vi "ProdaNG.TestValues.Get.vi"(8 "error in (no error)":errorcluster, 10 "testStepId":i32, 11 "dbHandleIn":i32) -> (0 "error out":errorcluster, 2 "TestStepValues":T1[](array[typedef]) {"minimum" format="%#.3f"; "maximum" format="%#.3f"}, 3 "dbHandle":i32)   [LabVIEW 2016]
doc: "This function returns a product structure for a product, which is identified by a part and a serial number.\nImportant information: The field 'individual' was taken over from the field 'allgemein' of the legacy data directly. Because of this most products have the value 0 further on and only a few the value 1. \nParameter:\nhandle is an Integer, which is returned by the function Login() at the creation of a new connection.\nwabcoPartId is the Id of the part.\nserialNumber is the serial number of the product for the part above.\nproduct is a pointer on a product structure, which is filled if the returncode is 0. The structure must be defined in the calling program.\n\nReturncodes:\n0 No error\n< 0 ORACLE Error code\n6 (ERROR_INVALID_HANDLE) in case of an invalid handle\n1403 Record does not exist"
uses:
  Controls/ProdaNG.TestValue.ctl
  Controls/ProdaNG.TestValueSize.ctl
  <vilib>/Utility/importsl/GetValueByPointer/datatype.ctl
  <vilib>/Utility/importsl/GetValueByPointer/GetValueByPointer.xnode
  prodllNG.dll
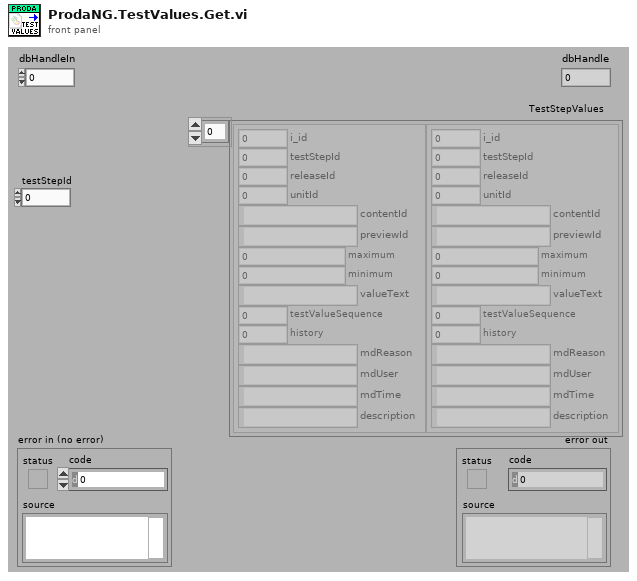
[diagram p1: front panel]
types:
  T1 = typedef "ProdaNG.TestValue.ctl" = cluster{"i_id":i32, "testStepId":i32, "releaseId":i32, "unitId":i32, "contentId":string, "previewId":string, "maximum":dbl, "minimum":dbl, "valueText":string, "testValueSequence":i32, "history":i32, "mdReason":string, "mdUser":string, "mdTime":string, "description":string}
  T2 = typedef "ProdaNG.TestValueSize.ctl" = cluster{"i_id":i32, "testStepId":i32, "releaseId":i32, "unitId":i32, "contentId":i32, "previewId":i32, "maximum":i32, "minimum":i32, "valueText":i32, "testValueSequence":i32, "history":i32, "mdReason":i32, "mdUser":i32, "mdTime":i32, "description":i32}
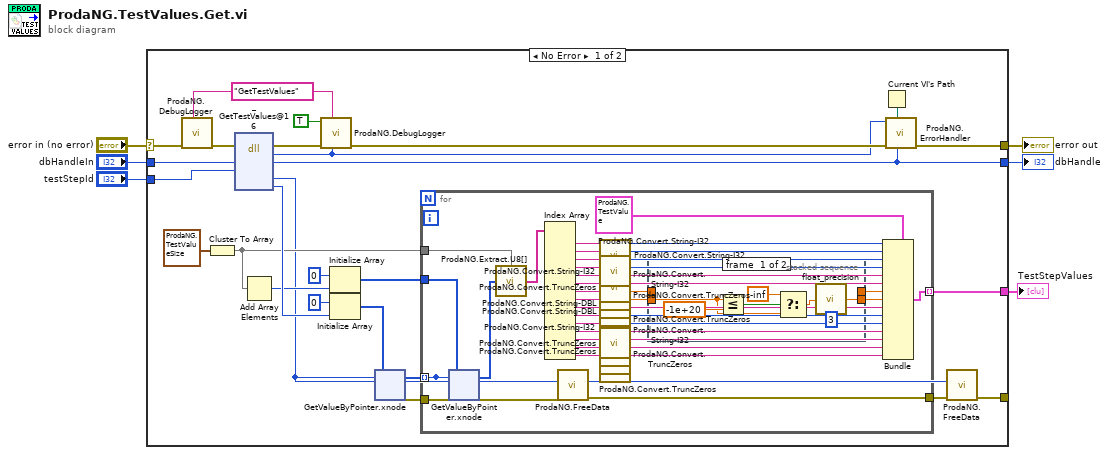
[diagram p0: block diagram]
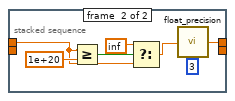
[diagram p2: hidden frame]
diagram:
  n1 = case shown="No Error" "error in (no error)" {
    selector: "error in (no error)" -> [w27 w120]
    tunnel: [w32 w120] -> w5
    tunnel: "dbHandleIn" -> [w29 w119]
    tunnel: [w30 w119] -> w3
    tunnel: "testStepId" -> [w14 _]
    tunnel: [w11 _] -> w1
    tunnel: [w9 _] -> _
    frame No Error {
      w23 = "GetTestValues" ("cmd")
      n2 = call "ProdaNG.DebugLogger.vi"("cmd"=w23, "error in (no error)"=w27) -> ("error out"=w26:errorcluster)  [unwired: 9 in]
      n3 = Cluster To Array(cluster=T2 {"i_id"=4, "testStepId"=4, "releaseId"=4, "unitId"=4, "contentId"=16, "previewId"=16, "maximum"=8, "minimum"=8, "valueText"=258, "testValueSequence"=4, "history"=4, "mdReason"=514, "mdUser"=22, "mdTime"=24, "description"=514} ("TestStepValueSize")) -> (array=w12:i32[])
      n4 = dll-call lib="D:/Maszup/WABCO/SVN/LineTraceSystem/SOFTWARE/sources/Database/ProdaNG/prodllNG.dll" fn="_GetTestValues@16" ("ProDLL wrapper.dll:ProDLL_wrapper_GetWabcoParts_GetData")(error in=w26, "dbHandle"=w29, "testStepId"=w14) -> (error out=w25:errorcluster, "return type"=w22:i32, "dbHandle"=w30:i32, "testValues"=w8:u32, "countPtr"=w17:i32)  [unwired: 5 in, 1 out]
      n5 = Add Array Elements(numeric array=w12) -> (sum=w13:i32)
      n6 = call "ProdaNG.DebugLogger.vi"("return type"=w22, "cmd"=w23, "error in (no error)"=w25, "done? (F)"=TRUE) -> ("error out"=w24:errorcluster)  [unwired: 7 in]
      n7 = Initialize Array(u8 0 ("element"), w13) -> (w15:u8[])
      n8 = Initialize Array(u32 0 ("element"), w17) -> (w21:u32[])
      n9 = xnode "GetValueByPointer.xnode"("Pointer"=w8, "InputType"=w21) -> ("Output"=w18:u32[], "ErrorOut"=w19:errorcluster)  [unwired: 2 in]
      n10 = for {
        tunnel: w19 -> [w74]
        tunnel: w18 -> [w42] mode=indexing
        tunnel: w15 -> [w73]
        tunnel: w12 -> [w57]
        tunnel: [w56] -> w11 mode=indexing
        tunnel: [w41] -> w10
        n11 = xnode "GetValueByPointer.xnode"("Pointer"=w42, "InputType"=w73, "ErrorIn"=w74) -> ("Output"=w59:u8[], "ErrorOut"=w43:errorcluster)  [unwired: 1 in]
        n12 = call "ProdaNG.Extract.U8[].vi"("unsigned byte array"=w59, "Sizes"=w57) -> ("Elements"=w58:string[])
        n13 = Index Array(array=w58) -> (element #1=w61:string, element #2=w60:string, element #3=w71:string, element #4=w68:string, element #5=w65:string, element #6=w67:string, element #7=w55:string, element #8=w54:string, element #9=w53:string, element #10=w51:string, element #11=w49:string, element #12=w47:string, element #13=w44:string, element #14=w38:string, element #15=w37:string)  [unwired: 15 in]
        n14 = call "ProdaNG.FreeData.vi"("error in (no error)"=w43, "Pointers"=w42) -> ("error out"=w41:errorcluster)  [unwired: 9 in]
        n15 = call "ProdaNG.Convert.String-I32.vi"("unsigned byte string"=w61) -> ("32bit integer"=w63:i32)  [unwired: 10 in]
        n16 = call "ProdaNG.Convert.String-I32.vi"("unsigned byte string"=w60) -> ("32bit integer"=w62:i32)  [unwired: 10 in]
        n17 = call "ProdaNG.Convert.String-I32.vi"("unsigned byte string"=w71) -> ("32bit integer"=w70:i32)  [unwired: 10 in]
        n18 = call "ProdaNG.Convert.String-I32.vi"("unsigned byte string"=w68) -> ("32bit integer"=w69:i32)  [unwired: 10 in]
        n19 = call "ProdaNG.Convert.TruncZeros.vi"("string with \\0s"=w65) -> ("LV string"=w64:string)  [unwired: 10 in]
        n20 = call "ProdaNG.Convert.TruncZeros.vi"("string with \\0s"=w67) -> ("LV string"=w66:string)  [unwired: 10 in]
        n21 = call "ProdaNG.Convert.String-DBL.vi"("unsigned byte string"=w55) -> ("dbl integer"=w33:dbl)  [unwired: 10 in]
        n22 = call "ProdaNG.Convert.String-DBL.vi"("unsigned byte string"=w54) -> ("dbl integer"=w36:dbl)  [unwired: 10 in]
        n23 = call "ProdaNG.Convert.TruncZeros.vi"("string with \\0s"=w53) -> ("LV string"=w52:string)  [unwired: 10 in]
        n24 = call "ProdaNG.Convert.String-I32.vi"("unsigned byte string"=w51) -> ("32bit integer"=w50:i32)  [unwired: 10 in]
        n25 = call "ProdaNG.Convert.String-I32.vi"("unsigned byte string"=w49) -> ("32bit integer"=w48:i32)  [unwired: 10 in]
        n26 = call "ProdaNG.Convert.TruncZeros.vi"("string with \\0s"=w47) -> ("LV string"=w46:string)  [unwired: 10 in]
        n27 = call "ProdaNG.Convert.TruncZeros.vi"("string with \\0s"=w44) -> ("LV string"=w45:string)  [unwired: 10 in]
        n28 = call "ProdaNG.Convert.TruncZeros.vi"("string with \\0s"=w38) -> ("LV string"=w40:string)  [unwired: 10 in]
        n29 = call "ProdaNG.Convert.TruncZeros.vi"("string with \\0s"=w37) -> ("LV string"=w39:string)  [unwired: 10 in]
        n30 = stacked-sequence {
          tunnel: w36 -> [w78 _]
          tunnel: [w76 _] -> w35
          tunnel: [_ w84] -> w34
          tunnel: w33 -> [_ w85]
          frame #0 {
            n31 = Less Or Equal?(x=w78, y=-1e+20) -> (x <= y?=w81:bool)
            n32 = Select(t=-inf, s=w81, f=w78) -> (s? t:f=w75:dbl)
            n33 = call "float_precision.vi"("input"=w75, "precision"=3) -> ("output"=w76:dbl)
          }
          frame #1 {
            n34 = Greater Or Equal?(x=w85, y=1e+20) -> (x >= y?=w88:bool)
            n35 = Select(t=inf, s=w88, f=w85) -> (s? t:f=w83:dbl)
            n36 = call "float_precision.vi"("input"=w83, "precision"=3) -> ("output"=w84:dbl)
          }
        }
        n37 = Bundle(cluster=T1 {"i_id"=0, "testStepId"=0, "releaseId"=0, "unitId"=0, "contentId"="", "previewId"="", "maximum"=0.0, "minimum"=0.0, "valueText"="", "testValueSequence"=0, "history"=0, "mdReason"="", "mdUser"="", "mdTime"="", "description"=""} ("TestValue"), "i_id"=w63, "testStepId"=w62, "releaseId"=w70, "unitId"=w69, "contentId"=w64, "previewId"=w66, "maximum"=w34, "minimum"=w35, "valueText"=w52, "testValueSequence"=w50, "history"=w48, "mdReason"=w46, "mdUser"=w45, "mdTime"=w40, "description"=w39) -> (w56:T1)
      }
      n38 = Current VI's Path() -> (path=w31:path)
      n39 = call "ProdaNG.ErrorHandler.vi"("dbHandleIn"=w30, "Path"=w31, "error in"=w24, "output_parameter"=w22) -> ("error out"=w32:errorcluster)  [unwired: 7 in]
      n40 = call "ProdaNG.FreeData.vi"("error in (no error)"=w10, "Pointers"=w8) -> ("error out"=w9:errorcluster)  [unwired: 9 in]
    }
    frame Error {
    }
  }
  "error out" <- w5
  "dbHandle" <- w3
  "TestStepValues" <- w1
